vi "Build Entity Info.vi"(10 "Entity":refnum<class "Entity.lvclass">) -> (2 "Entity Info":T1)   [LabVIEW 2020, in "Conditu2.lvlib" / "Entity Manager.lvclass"]
uses:
  Entity Manager.lvclass
  Entity/Entity.lvclass
  Entity Info.ctl
  Columns/Type/Type.lvclass
  Field Type.ctl
  Columns/Type/Type.lvclass/Type.ctl
  <vilib>/Utility/LVClass/Get LV Class Name.vi
  Conditu2.lvlib
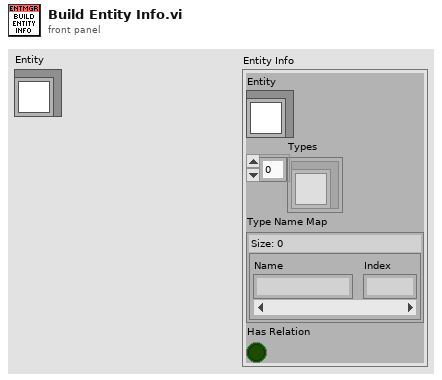
[diagram p1: front panel]
types:
  T1 = typedef "Conditu2.lvlib/Entity Manager.lvclass/Entity Info.ctl" = cluster{"Entity":refnum<class "Entity.lvclass">, "Types":refnum<class "Type.lvclass">[], "Type Name Map":map{string, i32}, "Has Relation":bool}
  T2 = typedef "Conditu2.lvlib/Field Type.ctl" = enum16{"None", "ID", "Boolean", "Integer", "Double", "Timestamp", "String", "Text", "Entity"}
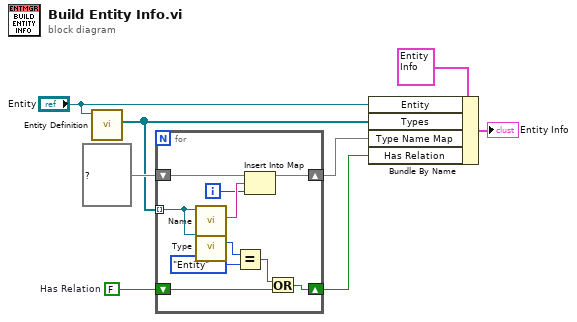
[diagram p0: block diagram]
diagram:
  w3 = FALSE  # Has Relation
  n1 = call "Entity Definition.vi"("Entity in"="Entity") -> ("Definition"=w5:refnum<class "Type.lvclass">[])  [unwired: 10 in]
  n2 = for {
    tunnel: w5 -> [w14] mode=indexing
    shift-right: [w15] -> w6
    shift-left: map{string, i32} {} ("Type Name Map") -> [w18]
    shift-right: [w9] -> w2
    shift-left: w3 -> [w11]
    i -> [w16]
    n3 = call "Name.vi"("Type in"=w14) -> ("Table Name"=w17:string)  [unwired: 10 in]
    n4 = call "Type.vi"("Type in"=w14) -> ("Type"=w13:T2)  [unwired: 10 in]
    n5 = Equal?(x=w13, y=Field_Type."Entity") -> (x = y?=w10:bool)
    n6 = Insert Into Map(map in=w18, key=w17, value=w16) -> (map out=w15:map{string, i32})  [unwired: 2 out]
    n7 = Or(x=w10, y=w11) -> (x .or. y?=w9:bool)
  }
  n8 = Bundle By Name(cluster=T1 {"Entity"=refnum, "Types"=[], "Type Name Map"={}, "Has Relation"=FALSE} ("Known Entity"), "Entity"="Entity", "Types"=w5, "Type Name Map"=w6, "Has Relation"=w2) -> (→"Entity Info":T1)
